vi "write_settings.vi"(4 "Zone 1 SP":dbl, 5 "Zone 3 SP":dbl, 6 "Notes":string, 7 "Zone 2 SP":dbl, 8 "error in":errorcluster, 9 "Zone 3 PID":T1={"proportional gain (Kc)"=1.0, "integral time (Ti, min)"=0.01, "derivative time (Td, min)"=0.0} {"derivative time (Td, min)" format="%.3f"; "integral time (Ti, min)" format="%.3f"; "proportional gain (Kc)" format="%.3f"}, 10 "Zone 2 PID":T1={"proportional gain (Kc)"=1.0, "integral time (Ti, min)"=0.01, "derivative time (Td, min)"=0.0} {"derivative time (Td, min)" format="%.3f"; "integral time (Ti, min)" format="%.3f"; "proportional gain (Kc)" format="%.3f"}, 11 "Zone 1 PID":T1={"proportional gain (Kc)"=1.0, "integral time (Ti, min)"=0.01, "derivative time (Td, min)"=0.0} {"derivative time (Td, min)" format="%.3f"; "integral time (Ti, min)" format="%.3f"; "proportional gain (Kc)" format="%.3f"}) -> (0 "error out":errorcluster)   [LabVIEW 2020]
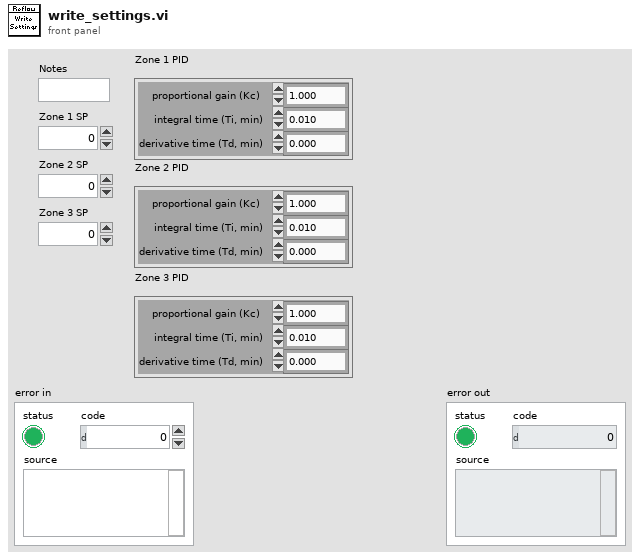
[diagram p1: front panel]
types:
  T1 = cluster{"proportional gain (Kc)":dbl, "integral time (Ti, min)":dbl, "derivative time (Td, min)":dbl}
  T2 = enum16{"open", "replace", "create", "open or create", "replace or create", "replace or create with confirmation"}
  T3 = cluster{"Notes":string, "Zone 1 SP":dbl, "Zone 2 SP":dbl, "Zone 3 SP":dbl, "Zone 1 PID":cluster{"proportional gain (Kc)":dbl, "integral time (Ti, min)":dbl, "derivative time (Td, min)":dbl}, "Zone 2 PID":cluster{"proportional gain (Kc)":dbl, "integral time (Ti, min)":dbl, "derivative time (Td, min)":dbl}, "Zone 3 PID":cluster{"proportional gain (Kc)":dbl, "integral time (Ti, min)":dbl, "derivative time (Td, min)":dbl}}
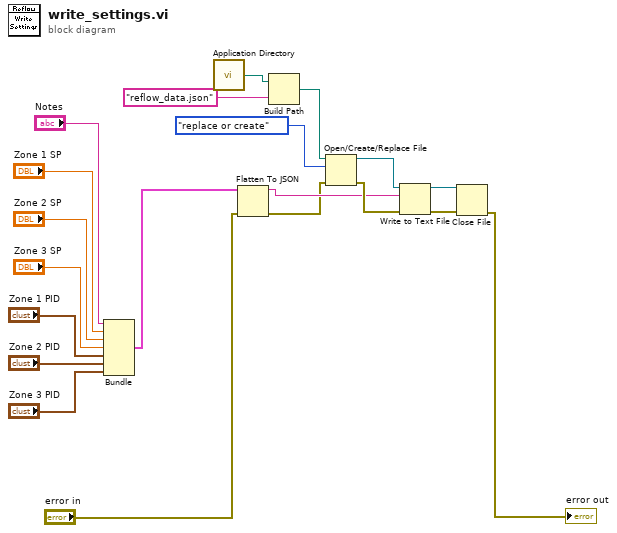
[diagram p0: block diagram]
diagram:
  n1 = Bundle("Notes"="Notes", "Zone 1 SP"="Zone 1 SP", "Zone 2 SP"="Zone 2 SP", "Zone 3 SP"="Zone 3 SP", "Zone 1 PID"="Zone 1 PID", "Zone 2 PID"="Zone 2 PID", "Zone 3 PID"="Zone 3 PID") -> (w13:T3)  [unwired: 1 in]
  n2 = call <vilib>:"Application Directory.vi"() -> ("Application Directory"=w10:path)
  n3 = Flatten To JSON(anything=w13, error in (no error)="error in") -> (JSON string=w2:string, 11:w1:errorcluster)  [unwired: 1 in]
  n4 = Build Path(base path=w10, name or relative path="reflow_data.json") -> (appended path=w8:path)
  n5 = Open/Create/Replace File(file path (use dialog)=w8, error in=w1, operation (0:open)=T2."replace or create") -> (refnum out=w6:refnum<file>, error out=w7:errorcluster)  [unwired: 3 in, 1 out]
  n6 = Write to Text File(file (use dialog)=w6, text=w2, error in=w7) -> (refnum out=w4:refnum<file>, error out=w5:errorcluster)  [unwired: 1 in, 1 out]
  n7 = Close File(refnum=w4, error in=w5) -> (error out=→"error out":errorcluster)  [unwired: 1 out]
